vi "5.1 CSM API String to Array.vi"() -> ()   [LabVIEW 2017]
doc: "#### Overview\n\nDemonstrates API String support for array types.\n\n#### Introduction\n\nIn the API String definition for Arrays, comma (`,`) is used for element separation, semicolon (`;`) is used for row separation, and brackets (`[` and `]`) are used as boundary symbols. For non-complex mixed data types, brackets can be omitted.\n\n**Examples:**\n\n- `a,b,c,d,e`, `[a,b,c,d,e]`, and `[a;b;c;d;e]` all represent an array containing 5 elements.\n- `a1, b1, c1, d1, e1; a2, b2, c2, d2, e2` and `[a1, b1, c1, d1, e1; a2, b2, c2, d2, e2]` represent a 2x5 2D array.\n\n**Special Case Note:**\n\n- An empty string converts to prototype input value.\n\n#### Steps\n\n- step1: Empty string converts to prototype input value.\n- step2: 1D array conversion.\n- step3: 2D array conversion."
uses:
  2002176a-b278-42b8-8ff5-87e066bf117a.vi
  3a5d3adc-f18e-4b24-90ad-4b548b3d9b49.vi
  86d59eec-a28c-42d3-be80-1aa62744661d.vi
  addons/API-String-Arugments-Support/_Support/Convert API String Arguments to Data(variant).vi
panel:
  out "Retrieve Array 3":T1={"Empty API String"="", "1D DBL"=[[3.12, 4.11, 5.0], [2.0, 3.0, 4.0]], "Retrieved Data"=[[3.12, 4.11, 5.0]]}
  out "Retrieve Array 2":T2={"Empty API String"="", "1D DBL"=[3.12, 4.11, 5.0], "Retrieved Data"=[3.12, 4.11, 5.0]}
  out "Retrieve Array 1":T2={"Empty API String"="", "1D DBL"=[3.12, 4.11, 5.0], "Retrieved Data"=[3.12, 4.11, 5.0]}
  # "#CSM-Example Overview\n\nDemonstrates API String support for array types."
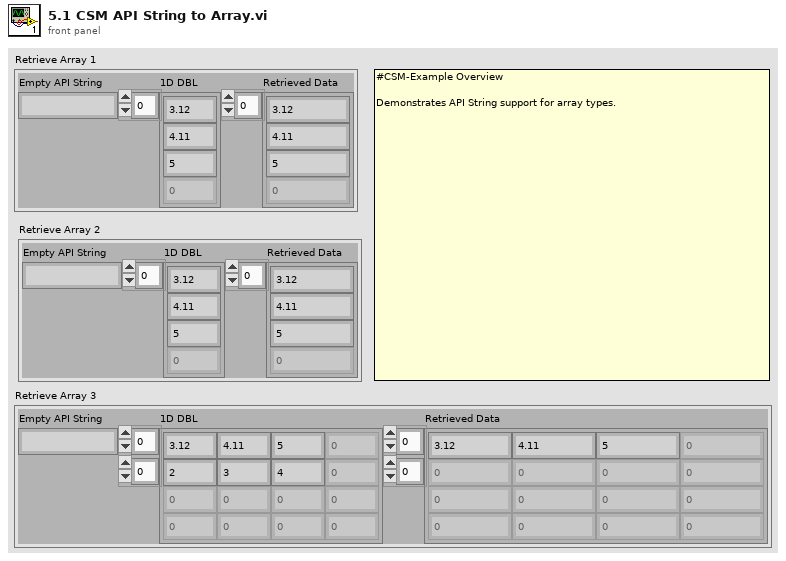
[diagram p1: front panel]
types:
  T1 = cluster{"Empty API String":string, "1D DBL":dbl[][], "Retrieved Data":dbl[][]}
  T2 = cluster{"Empty API String":string, "1D DBL":dbl[], "Retrieved Data":dbl[]}
  T3 = cluster{"String":string, "Data 4":dbl[], "Data":dbl[]}
  T4 = cluster{"String":string, "Data 4":dbl[][], "Data":dbl[][]}
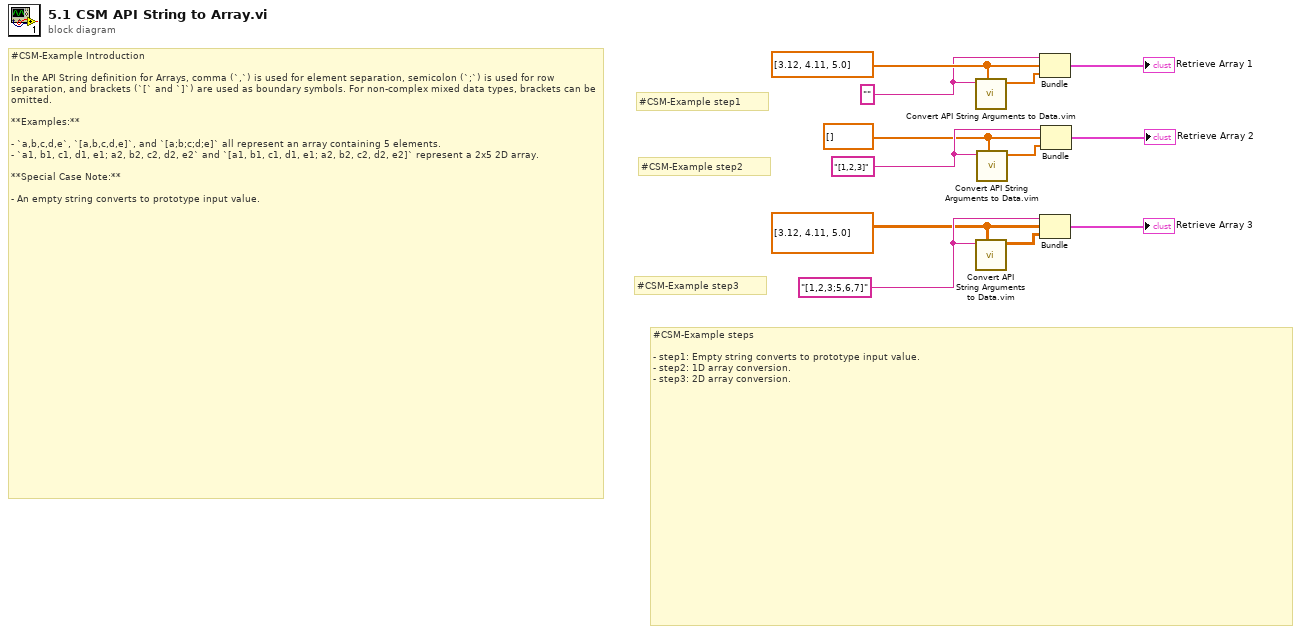
[diagram p0: block diagram]
diagram:
  w4 = "[1,2,3;5,6,7]" ("String")
  w2 = dbl[][] [[3.12, 4.11, 5.0]] ("Data 4")
  w8 = "[1,2,3]" ("String")
  w6 = dbl[] [] ("Data 4")
  w9 = "" ("String")
  w11 = dbl[] [3.12, 4.11, 5.0] ("Data 4")
  # "#CSM-Example steps\n\n- step1: Empty string converts to prototype input value.\n- step2: 1D array conversion.\n- step3: 2D array conversion."
  # "#CSM-Example step3"
  # "#CSM-Example step2"
  # "#CSM-Example step1"
  # "#CSM-Example Introduction\n\nIn the API String definition for Arrays, comma (`,`) is used for element separation, semicolon (`;`) is used for row separation, and brackets (`[` and `]`) are used as boundary symbols. For non-complex mixed data types, brackets can be omitted.\n\n**Examples:**\n\n- `a,b,c,d,e`, `[a,b,c,d,e]`, and `[a;b;c;d;e]` all represent an array containing 5 elements.\n- `a1, b1, c1, d1, e1; a2, b2, c2, d2, e2` and `[a1, b1, c1, d1, e1; a2, b2, c2, d2, e2]` represent a 2x5 2D array.\n\n**Special Case Note:**\n\n- An empty string converts to prototype input value."
  n1 = call "Convert API String Arguments to Data.vim"("Reference Type"=w11, "API String"=w9) -> ("Data"=w12:dbl[])  [unwired: 6 in, 1 out]
  n2 = call "Convert API String Arguments to Data.vim"("Reference Type"=w2, "API String"=w4) -> ("Data"=w1:dbl[][])  [unwired: 6 in, 1 out]
  n3 = call "Convert API String Arguments to Data.vim"("Reference Type"=w6, "API String"=w8) -> ("Data"=w5:dbl[])  [unwired: 6 in, 1 out]
  n4 = Bundle("String"=w9, "Data 4"=w11, "Data"=w12) -> (→"Retrieve Array 1":T3)  [unwired: 1 in]
  n5 = Bundle("String"=w4, "Data 4"=w2, "Data"=w1) -> (→"Retrieve Array 3":T4)  [unwired: 1 in]
  n6 = Bundle("String"=w8, "Data 4"=w6, "Data"=w5) -> (→"Retrieve Array 2":T3)  [unwired: 1 in]
